vi "Write modulationConfig.vi"(8 "error in (no error)":errorcluster, 10 "modulationConfig":T1 {"modulationRate" format="%#_6p"; "Deadband" format="%#_6p"; "SwitchingSpeed" format="%#_6p"}, 11 "BuckBoost configuration in":refnum<class "BuckBoost configuration.lvclass">) -> (0 "error out":errorcluster, 3 "BuckBoost configuration out":refnum<class "BuckBoost configuration.lvclass">)   [LabVIEW 2017, in "BuckBoost configuration.lvclass"]
uses:
  BuckBoost configuration.lvclass
  <vilib>/NI/PowerElectronicsControl/Buck-Boost/RealTime/modulationConfig.ctl
  BuckBoost configuration.lvclass/BuckBoost configuration.ctl
  <vilib>/NI/PowerElectronicsControl/Buck-Boost/RealTime/BuckBoostInterface.lvlib
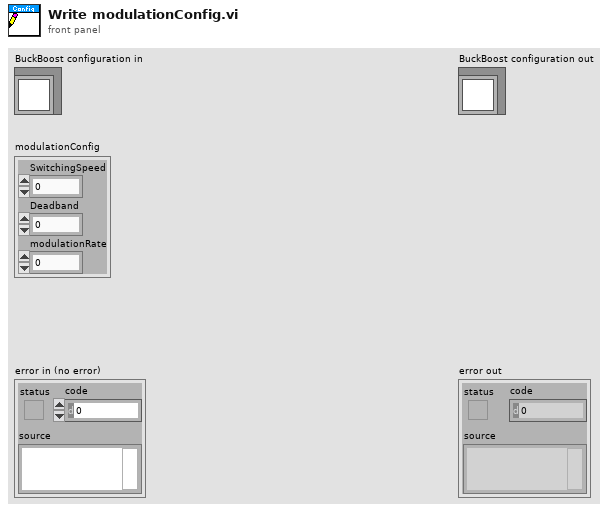
[diagram p1: front panel]
types:
  T1 = typedef "BuckBoostInterface.lvlib/modulationConfig.ctl" = cluster{"SwitchingSpeed":dbl, "Deadband":dbl, "modulationRate":dbl}
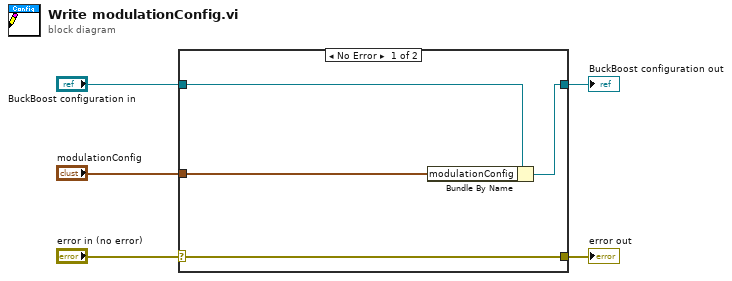
[diagram p0: block diagram]
diagram:
  n1 = case shown="No Error" "error in (no error)" {
    selector: "error in (no error)" -> [w9 w10]
    tunnel: [w9 w10] -> w4
    tunnel: [w7 w11] -> w2
    tunnel: "BuckBoost configuration in" -> [w8 w11]
    tunnel: "modulationConfig" -> [w6 _]
    frame No Error {
      n2 = Bundle By Name(cluster=w8, "modulationConfig"=w6) -> (w7:refnum<class "BuckBoost configuration.lvclass">)
    }
    frame Error {
    }
  }
  "error out" <- w4
  "BuckBoost configuration out" <- w2
